vi "Initialize MUX Register.vi"(7 "# of Injectors":u8, 8 "error in (no error)":errorcluster, 10 "Name":string, 11 "FPGA Ref":refnum<k20>) -> (0 "error out":errorcluster, 3 "FPGA Ref out":refnum<k20>)   [LabVIEW 2019, in "Fuel Injector Analysis Addon Engine.lvlib"]
uses:
  Fuel Injector Analysis Addon Engine.lvlib
  <vilib>/NI/LVFPGA Adv Session Resources/OpenByNameSubVI.vi
  <vilib>/rvi/interface/common/dynamic/niFpgaEscapeDelimiterAndNull.vi
  <vilib>/Utility/error.llb/Error Cluster From Error Code.vi
  <vilib>/rvi/errors/niLvFpgaAdjustHostInterfaceError.vi
  <vilib>/FPGAPlugInAG/Dynamic/niLvFpga_Close_Dynamic.vi
  <vilib>/NI/LVFPGA Adv Session Resources/OpenByName.xnode
  <vilib>/rvi/interface/nirviReadWriteControl/nirviReadWriteControl.xnode
  <vilib>/rvi/interface/nirviCloseFPGA/nirviCloseFPGA.xnode
  <vilib>/rvi/interface/Simulation/niFpgaSimulationCallBeginRW.vi
  NiFpgaLv.dll
  <vilib>/NI/LVFPGA Adv Session Resources/LVFPGAAdvSessionResources.lvlib
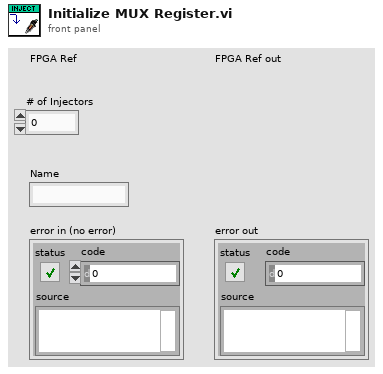
[diagram p1: front panel]
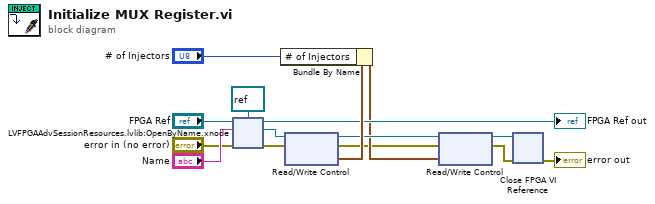
[diagram p0: block diagram]
diagram:
  n1 = xnode "LVFPGAAdvSessionResources.lvlib:OpenByName.xnode"("FPGA VI Reference in"="FPGA Ref", "Resource name in"="Name", "Single resource reference type in"=refnum<k20> refnum ("Injector.MUX.Setting"), "Error in"="error in (no error)") -> ("Single resource reference out"=w6:refnum<k20>, "Error out"=w7:errorcluster, "FPGA VI Reference out"=→"FPGA Ref out":refnum<k20>)
  n2 = xnode "Read/Write Control"("FPGA VI Reference In"=w6, "error in"=w7) -> ("FPGA VI Reference Out"=w5:refnum<k20>, "error out"=w1:errorcluster, "Value"=w15:cluster{"# of Injectors":u8})
  n3 = Bundle By Name(cluster=w15, "# of Injectors"="# of Injectors") -> (w2:cluster{"# of Injectors":u8})
  n4 = xnode "Read/Write Control"("FPGA VI Reference In"=w5, "error in"=w1, "Value"=w2) -> ("FPGA VI Reference Out"=w12:refnum<k20>, "error out"=w13:errorcluster)
  n5 = xnode "Close FPGA VI Reference"("FPGA VI Reference In"=w12, "error in"=w13) -> ("error out"=→"error out":errorcluster)
